vi "Create and Destroy.vi"(8 "Error In":errorcluster) -> (0 "Error Out":errorcluster)   [LabVIEW 2017, in "Tests.lvlib" / "Writer.lvlib"]
uses:
  Writer.lvlib
  src/LabPack/Public/Writer/Writer.lvclass
  <vilib>/addons/_JKI Toolkits/Caraya/classes/Test/Test.lvclass
  <vilib>/addons/_JKI Toolkits/Caraya/classes/Assert/Assert.lvclass
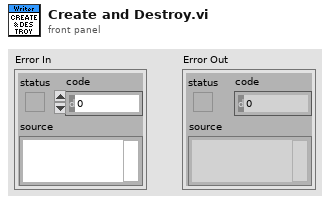
[diagram p1: front panel]
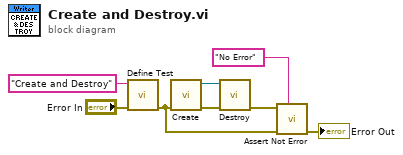
[diagram p0: block diagram]
diagram:
  n1 = call <vilib>:"Define Test.vi"("error in (no error)"="Error In", "Label (VI Title)"="Create and Destroy") -> ("error out"=w4:errorcluster)  [unwired: 9 in]
  n2 = call "Create.vi"("Error In"=w4) -> ("Error Out"=w7:errorcluster, "Writer"=w8:refnum<class "Writer.lvclass">)  [unwired: 9 in]
  n3 = call "Destroy.vi"("Error In"=w7, "Writer"=w8) -> ("Error Out"=w3:errorcluster)  [unwired: 9 in]
  n4 = call <vilib>:"Assert Not Error.vi"("Label"="No Error", "error in (no error)"=w4, "Not Error?"=w3) -> ("error out"=→"Error Out":errorcluster)  [unwired: 8 in]
